vi "Lab Panel V4.87.vi"() -> ()   [LabVIEW 2013] (continued)
                          }
                          frame #9 {
                            n2885 = Greater?(x=w5378, y=w5381) -> (0:w5380:bool)
                            n2886 = case shown="True" w5380 {
                              tunnel: [w5382 0] -> w5377
                              tunnel: w5378 -> [w5382 _]
                              tunnel: w5379 -> [_ w5383]
                              frame False {
                              }
                              frame True {
                                n2887 = Concatenate Strings("LA05-2 ", w5383) -> (w5386:string)
                                n2888 = One Button Dialog(message=w5386) -> ()  [unwired: 1 in, 1 out]
                              }
                            }
                          }
                        }
                        n2889 = Bundle By Name(cluster=w5285, "LAB01-1"=w5283, "LAB01-2"=w5281, "LAB02-1"=w5278, "LAB02-2"=w5275, "LAB03-1"=w5273, "LAB03-2"=w5272, "LAB04-1"=w5269, "LAB04-2"=w5267, "LAB05-1"=w5265, "LAB05-2"=w5263) -> (w5284:T8)
                        n2890 = local write "JIG RELAY CYCLES"(w5284) -> ()
                      }
                    }
                  }
                }
              }
            }
          }
          frame #19 {
            # "get temperature values"
            n2891 = local read "PANEL #"() -> (w5387:dbl)
            n2892 = local read "simulate"() -> (w5400:bool)
            n2893 = local read "Temp Test Cal"() -> (w5397:dbl)
            n2894 = stacked-sequence {
              seq-local: [w5401 _] -> [_ w5439]
              tunnel: w5400 -> [_ w5453]
              tunnel: T14 {"1  (A) cal"=1.0, "1 (V) cal"=1.0, "1 (PF) cal"=1.0, "1 (TL) cal"=1.0, "1 (TN) cal"=1.0, "2 (A) cal"=1.0, "2 (V) cal"=1.0, "2 (PF) cal"=1.0, "2 (TL) cal"=1.0, "2 (TN) cal"=1.0} ("CAL LAB01") -> [_ w5452]
              tunnel: w5398 -> [_ w5451]
              tunnel: w5397 -> [_ w5450]
              tunnel: w5396 -> [_ w5449]
              tunnel: w5395 -> [_ w5448]
              tunnel: w5394 -> [_ w5447]
              tunnel: w5393 -> [_ w5446]
              tunnel: w5392 -> [_ w5445]
              tunnel: w5391 -> [_ w5444]
              tunnel: w5390 -> [_ w5443]
              tunnel: w5389 -> [_ w5442]
              tunnel: w5388 -> [_ w5441]
              tunnel: w5387 -> [_ w5440]
              frame #0 {
                n2895 = local read "Select COM port"() -> (w5404:refnum<visa-resource-name>)
                "COM port" <- w5404
                n2896 = global write "Global 1.vi" "tmp dly lps"("Temp Delay Lps") -> ()
                n2897 = global write "Global 1.vi" "dly value"("Temp Value") -> ()
                n2898 = global write "Global 1.vi" "COM port"(w5404) -> ()
                n2899 = local read "jig cycle"() -> (w5406:dbl)
                n2900 = local read "on loops"() -> (w5408:dbl)
                n2901 = Add(x=w5408, y=3) -> (x+y=w5409:dbl)
                n2902 = local read "PANEL #"() -> (w5405:dbl)
                n2903 = Equal?(x=w5406, y=w5409) -> (x = y?=w5401:bool)
                n2904 = case shown="True" w5401 {
                  tunnel: w5405 -> [_ w5413]
                  frame False {
                  }
                  frame True {
                    n2905 = local read "simulate"() -> (w5410:bool)
                    n2906 = case shown="1" w5413 {
                      tunnel: 1.0 -> [_ w5418 w5420 w5426 w5430 w5435]
                      tunnel: w5410 -> [_ w5414 w5419 w5424 w5431 w5434]
                      frame 0, Default {
                      }
                      frame 1 {
                        w5416 = FALSE
                        n2907 = call "sub vi - GET ALL TEMP v6.vi"("LA01-EN"=TRUE, "simulate"=w5414, "LA02-EN"=w5416, "LA03-EN"=w5416, "LA04-EN"=w5416, "LA05-EN"=w5416, "Gen Cal Value"=w5418) -> ("LA01 TEMP"=w5415:T24)  [unwired: 3 in, 5 out]
                        n2908 = local write "LAB01 TEMP"(w5415) -> ()
                      }
                      frame 2 {
                        w5421 = FALSE
                        n2909 = call "sub vi - GET ALL TEMP v6.vi"("LA01-EN"=w5421, "simulate"=w5419, "LA02-EN"=TRUE, "LA03-EN"=w5421, "LA04-EN"=w5421, "LA05-EN"=w5421, "Gen Cal Value"=w5420) -> ("LA02 TEMP"=w5423:T24)  [unwired: 3 in, 5 out]
                        n2910 = local write "LAB02 TEMP"(w5423) -> ()
                      }
                      frame 3 {
                        w5427 = FALSE
                        n2911 = call "sub vi - GET ALL TEMP v6.vi"("LA01-EN"=w5427, "simulate"=w5424, "LA02-EN"=w5427, "LA03-EN"=TRUE, "LA04-EN"=w5427, "LA05-EN"=w5427, "Gen Cal Value"=w5426) -> ("LA03 TEMP"=w5425:T24)  [unwired: 3 in, 5 out]
                        n2912 = local write "LAB03 TEMP"(w5425) -> ()
                      }
                      frame 4 {
                        w5432 = FALSE
                        n2913 = call "sub vi - GET ALL TEMP v6.vi"("LA01-EN"=w5432, "simulate"=w5431, "LA02-EN"=w5432, "LA03-EN"=w5432, "LA04-EN"=TRUE, "LA05-EN"=w5432, "Gen Cal Value"=w5430) -> ("LA04 TEMP"=w5429:T24)  [unwired: 3 in, 5 out]
                        n2914 = local write "LAB04 TEMP"(w5429) -> ()
                      }
                      frame 5 {
                        w5437 = FALSE
                        n2915 = call "sub vi - GET ALL TEMP v6.vi"("LA01-EN"=w5437, "simulate"=w5434, "LA02-EN"=w5437, "LA03-EN"=w5437, "LA04-EN"=w5437, "LA05-EN"=TRUE, "Gen Cal Value"=w5435) -> ("LA05 TEMP"=w5436:T24)  [unwired: 3 in, 5 out]
                        n2916 = local write "LAB05 TEMP"(w5436) -> ()
                      }
                    }
                    n2917 = local write "TEMP"(TRUE) -> ()
                  }
                }
              }
              frame #1 {
                n2918 = case shown="True" w5439 {
                  tunnel: w5453 -> [_ w5467]
                  tunnel: w5452 -> [_ w5466]
                  tunnel: w5451 -> [_ w5465]
                  tunnel: w5450 -> [_ w5464]
                  tunnel: w5449 -> [_ w5463]
                  tunnel: w5448 -> [_ w5462]
                  tunnel: w5447 -> [_ w5461]
                  tunnel: w5446 -> [_ w5460]
                  tunnel: w5445 -> [_ w5459]
                  tunnel: w5444 -> [_ w5458]
                  tunnel: w5443 -> [_ w5457]
                  tunnel: w5442 -> [_ w5456]
                  tunnel: w5441 -> [_ w5455]
                  tunnel: w5440 -> [_ w5454]
                  frame False {
                  }
                  frame True {
                    n2919 = case shown="1" w5454 {
                      tunnel: w5467 -> [_ w5480 w5525 w5570 w5615 w5660]
                      tunnel: w5466 -> [_ w5479 w5524 w5569 w5614 w5659]
                      tunnel: w5465 -> [_ w5477 _ _ _ _]
                      tunnel: w5464 -> [_ w5473 w5523 w5568 w5613 w5658]
                      tunnel: w5463 -> [_ w5468 _ _ _ _]
                      tunnel: w5462 -> [_ _ w5514 _ _ _]
                      tunnel: w5461 -> [_ _ w5513 _ _ _]
                      tunnel: w5460 -> [_ _ _ w5559 _ _]
                      tunnel: w5459 -> [_ _ _ w5558 _ _]
                      tunnel: w5458 -> [_ _ _ _ w5604 _]
                      tunnel: w5457 -> [_ _ _ _ w5603 _]
                      tunnel: w5456 -> [_ _ _ _ _ w5649]
                      tunnel: w5455 -> [_ _ _ _ _ w5648]
                      frame ..0 {
                      }
                      frame 1 {
                        n2920 = case shown="False" w5480 {
                          tunnel: [w5511 w5512] -> w5496
                          tunnel: w5479 -> [_ w5512]
                          frame False {
                            n2921 = local read "CAL LAB01"() -> (w5511:T14)
                          }
                          frame True {
                          }
                        }
                        n2922 = local read "LAB01 TEMP"() -> (w5486:T12)
                        n2923 = local read "TEMP LA01"() -> (w5487:T9)
                        n2924 = call "sub vi - temperature delay v2.vi"("temp values IN"=w5487, "temp signals"=w5486) -> ("T2-N"=w5482:dbl, "T2-L"=w5483:dbl, "T1-N"=w5484:dbl, "T1-L"=w5485:dbl, "temp values OUT"=w5481:T43)  [unwired: 5 in]
                        n2925 = Unbundle By Name(w5496) -> ("1 (TL) cal"=w5491:dbl, "1 (TN) cal"=w5490:dbl, "2 (TL) cal"=w5489:dbl, "2 (TN) cal"=w5488:dbl)  [unwired: 6 out]
                        n2926 = local write "TEMP LA01"(w5481) -> ()
                        n2927 = Multiply(x=w5485, y=w5491) -> (x*y=w5478:dbl)
                        n2928 = Multiply(x=w5484, y=w5490) -> (x*y=w5475:dbl)
                        n2929 = Multiply(x=w5483, y=w5489) -> (x*y=w5472:dbl)
                        n2930 = Multiply(x=w5482, y=w5488) -> (x*y=w5471:dbl)
                        n2931 = case shown="True" w5477 {
                          tunnel: w5478 -> [w5505 w5510]
                          tunnel: w5473 -> [_ w5508]
                          tunnel: [w5505 w5509] -> w5476
                          tunnel: w5475 -> [w5504 w5507]
                          tunnel: [w5504 w5506] -> w5474
                          frame False {
                          }
                          frame True {
                            n2932 = Multiply(x=w5508, y=w5507) -> (x*y=w5506:dbl)
                            n2933 = Multiply(x=w5508, y=w5510) -> (x*y=w5509:dbl)
                          }
                        }
                        n2934 = case shown="True" w5468 {
                          tunnel: w5472 -> [w5498 w5503]
                          tunnel: w5473 -> [_ w5501]
                          tunnel: [w5498 w5502] -> w5470
                          tunnel: w5471 -> [w5497 w5500]
                          tunnel: [w5497 w5499] -> w5469
                          frame False {
                          }
                          frame True {
                            n2935 = Multiply(x=w5501, y=w5500) -> (x*y=w5499:dbl)
                            n2936 = Multiply(x=w5501, y=w5503) -> (x*y=w5502:dbl)
                          }
                        }
                        n2937 = local read "SIG LAB01-2"() -> (w5493:T2)
                        n2938 = local read "SIG LAB01-1"() -> (w5495:T2)
                        n2939 = Bundle By Name(cluster=w5495, "Tmp Live"=w5476, "Tmp Neut"=w5474) -> (w5494:T2)
                        n2940 = Bundle By Name(cluster=w5493, "Tmp Live"=w5470, "Tmp Neut"=w5469) -> (w5492:T2)
                        n2941 = local write "SIG LAB01-1"(w5494) -> ()
                        n2942 = local write "SIG LAB01-2"(w5492) -> ()
                      }
                      frame 2 {
                        n2943 = case shown="True" w5525 {
                          tunnel: [w5556 w5557] -> w5541
                          tunnel: w5524 -> [_ w5557]
                          frame False {
                            n2944 = local read "CAL LAB02"() -> (w5556:T15)
                          }
                          frame True {
                          }
                        }
                        n2945 = local read "LAB02 TEMP"() -> (w5532:T12)
                        n2946 = local read "TEMP LA02"() -> (w5531:T9)
                        n2947 = call "sub vi - temperature delay v2.vi"("temp values IN"=w5531, "temp signals"=w5532) -> ("T2-N"=w5526:dbl, "T2-L"=w5527:dbl, "T1-N"=w5528:dbl, "T1-L"=w5529:dbl, "temp values OUT"=w5530:T43)  [unwired: 5 in]
                        n2948 = Unbundle By Name(w5541) -> ("1 (TL) cal"=w5536:dbl, "1 (TN) cal"=w5535:dbl, "2 (TL) cal"=w5534:dbl, "2 (TN) cal"=w5533:dbl)  [unwired: 6 out]
                        n2949 = local write "TEMP LA02"(w5530) -> ()
                        n2950 = Multiply(x=w5529, y=w5536) -> (x*y=w5522:dbl)
                        n2951 = Multiply(x=w5528, y=w5535) -> (x*y=w5521:dbl)
                        n2952 = Multiply(x=w5527, y=w5534) -> (x*y=w5518:dbl)
                        n2953 = Multiply(x=w5526, y=w5533) -> (x*y=w5517:dbl)
                        n2954 = case shown="True" w5514 {
                          tunnel: w5522 -> [w5550 w5555]
                          tunnel: w5523 -> [_ w5553]
                          tunnel: [w5550 w5554] -> w5520
                          tunnel: w5521 -> [w5549 w5552]
                          tunnel: [w5549 w5551] -> w5519
                          frame False {
                          }
                          frame True {
                            n2955 = Multiply(x=w5553, y=w5552) -> (x*y=w5551:dbl)
                            n2956 = Multiply(x=w5553, y=w5555) -> (x*y=w5554:dbl)
                          }
                        }
                        n2957 = case shown="True" w5513 {
                          tunnel: w5518 -> [w5543 w5548]
                          tunnel: w5523 -> [_ w5546]
                          tunnel: [w5543 w5547] -> w5516
                          tunnel: w5517 -> [w5542 w5545]
                          tunnel: [w5542 w5544] -> w5515
                          frame False {
                          }
                          frame True {
                            n2958 = Multiply(x=w5546, y=w5545) -> (x*y=w5544:dbl)
                            n2959 = Multiply(x=w5546, y=w5548) -> (x*y=w5547:dbl)
                          }
                        }
                        n2960 = local read "SIG LAB02-2"() -> (w5538:T2)
                        n2961 = local read "SIG LAB02-1"() -> (w5540:T2)
                        n2962 = Bundle By Name(cluster=w5540, "Tmp Live"=w5520, "Tmp Neut"=w5519) -> (w5539:T2)
                        n2963 = Bundle By Name(cluster=w5538, "Tmp Live"=w5516, "Tmp Neut"=w5515) -> (w5537:T2)
                        n2964 = local write "SIG LAB02-1"(w5539) -> ()
                        n2965 = local write "SIG LAB02-2"(w5537) -> ()
                      }
                      frame 3 {
                        n2966 = case shown="False" w5570 {
                          tunnel: [w5601 w5602] -> w5586
                          tunnel: w5569 -> [_ w5602]
                          frame False {
                            n2967 = local read "CAL LAB03"() -> (w5601:T14)
                          }
                          frame True {
                          }
                        }
                        n2968 = local read "TEMP LA03"() -> (w5576:T9)
                        n2969 = local read "LAB03 TEMP"() -> (w5577:T12)
                        n2970 = call "sub vi - temperature delay v2.vi"("temp values IN"=w5576, "temp signals"=w5577) -> ("T2-N"=w5571:dbl, "T2-L"=w5572:dbl, "T1-N"=w5573:dbl, "T1-L"=w5574:dbl, "temp values OUT"=w5575:T43)  [unwired: 5 in]
                        n2971 = Unbundle By Name(w5586) -> ("1 (TL) cal"=w5581:dbl, "1 (TN) cal"=w5580:dbl, "2 (TL) cal"=w5579:dbl, "2 (TN) cal"=w5578:dbl)  [unwired: 6 out]
                        n2972 = local write "TEMP LA03"(w5575) -> ()
                        n2973 = Multiply(x=w5574, y=w5581) -> (x*y=w5567:dbl)
                        n2974 = Multiply(x=w5573, y=w5580) -> (x*y=w5566:dbl)
                        n2975 = Multiply(x=w5572, y=w5579) -> (x*y=w5563:dbl)
                        n2976 = Multiply(x=w5571, y=w5578) -> (x*y=w5562:dbl)
                        n2977 = case shown="True" w5558 {
                          tunnel: w5563 -> [w5588 w5593]
                          tunnel: w5568 -> [_ w5591]
                          tunnel: [w5588 w5592] -> w5561
                          tunnel: w5562 -> [w5587 w5590]
                          tunnel: [w5587 w5589] -> w5560
                          frame False {
                          }
                          frame True {
                            n2978 = Multiply(x=w5591, y=w5590) -> (x*y=w5589:dbl)
                            n2979 = Multiply(x=w5591, y=w5593) -> (x*y=w5592:dbl)
                          }
                        }
                        n2980 = case shown="True" w5559 {
                          tunnel: w5567 -> [w5595 w5600]
                          tunnel: w5568 -> [_ w5598]
                          tunnel: [w5595 w5599] -> w5565
                          tunnel: w5566 -> [w5594 w5597]
                          tunnel: [w5594 w5596] -> w5564
                          frame False {
                          }
                          frame True {
                            n2981 = Multiply(x=w5598, y=w5597) -> (x*y=w5596:dbl)
                            n2982 = Multiply(x=w5598, y=w5600) -> (x*y=w5599:dbl)
                          }
                        }
                        n2983 = local read "SIG LAB03-2"() -> (w5583:T2)
                        n2984 = local read "SIG LAB03-1"() -> (w5585:T2)
                        n2985 = Bundle By Name(cluster=w5585, "Tmp Live"=w5565, "Tmp Neut"=w5564) -> (w5584:T2)
                        n2986 = Bundle By Name(cluster=w5583, "Tmp Live"=w5561, "Tmp Neut"=w5560) -> (w5582:T2)
                        n2987 = local write "SIG LAB03-1"(w5584) -> ()
                        n2988 = local write "SIG LAB03-2"(w5582) -> ()
                      }
                      frame 4 {
                        n2989 = case shown="False" w5615 {
                          tunnel: [w5646 w5647] -> w5631
                          tunnel: w5614 -> [_ w5647]
                          frame False {
                            n2990 = local read "CAL LAB04"() -> (w5646:T14)
                          }
                          frame True {
                          }
                        }
                        n2991 = local read "LAB04 TEMP"() -> (w5621:T12)
                        n2992 = local read "TEMP LA04"() -> (w5622:T9)
                        n2993 = call "sub vi - temperature delay v2.vi"("temp values IN"=w5622, "temp signals"=w5621) -> ("T2-N"=w5616:dbl, "T2-L"=w5617:dbl, "T1-N"=w5618:dbl, "T1-L"=w5619:dbl, "temp values OUT"=w5620:T43)  [unwired: 5 in]
                        n2994 = Unbundle By Name(w5631) -> ("1 (TL) cal"=w5626:dbl, "1 (TN) cal"=w5625:dbl, "2 (TL) cal"=w5624:dbl, "2 (TN) cal"=w5623:dbl)  [unwired: 6 out]
                        n2995 = local write "TEMP LA04"(w5620) -> ()
                        n2996 = Multiply(x=w5619, y=w5626) -> (x*y=w5612:dbl)
                        n2997 = Multiply(x=w5618, y=w5625) -> (x*y=w5611:dbl)
                        n2998 = Multiply(x=w5617, y=w5624) -> (x*y=w5608:dbl)
                        n2999 = Multiply(x=w5616, y=w5623) -> (x*y=w5607:dbl)
                        n3000 = case shown="True" w5603 {
                          tunnel: w5608 -> [w5633 w5638]
                          tunnel: w5613 -> [_ w5636]
                          tunnel: [w5633 w5637] -> w5606
                          tunnel: w5607 -> [w5632 w5635]
                          tunnel: [w5632 w5634] -> w5605
                          frame False {
                          }
                          frame True {
                            n3001 = Multiply(x=w5636, y=w5635) -> (x*y=w5634:dbl)
                            n3002 = Multiply(x=w5636, y=w5638) -> (x*y=w5637:dbl)
                          }
                        }
                        n3003 = case shown="True" w5604 {
                          tunnel: w5612 -> [w5640 w5645]
                          tunnel: w5613 -> [_ w5643]
                          tunnel: [w5640 w5644] -> w5610
                          tunnel: w5611 -> [w5639 w5642]
                          tunnel: [w5639 w5641] -> w5609
                          frame False {
                          }
                          frame True {
                            n3004 = Multiply(x=w5643, y=w5642) -> (x*y=w5641:dbl)
                            n3005 = Multiply(x=w5643, y=w5645) -> (x*y=w5644:dbl)
                          }
                        }
                        n3006 = local read "SIG LAB04-2"() -> (w5628:T2)
                        n3007 = local read "SIG LAB04-1"() -> (w5630:T2)
                        n3008 = Bundle By Name(cluster=w5630, "Tmp Live"=w5610, "Tmp Neut"=w5609) -> (w5629:T2)
                        n3009 = Bundle By Name(cluster=w5628, "Tmp Live"=w5606, "Tmp Neut"=w5605) -> (w5627:T2)
                        n3010 = local write "SIG LAB04-1"(w5629) -> ()
                        n3011 = local write "SIG LAB04-2"(w5627) -> ()
                      }
                      frame 5.. {
                        n3012 = case shown="False" w5660 {
                          tunnel: [w5691 w5692] -> w5676
                          tunnel: w5659 -> [_ w5692]
                          frame False {
                            n3013 = local read "CAL LAB05"() -> (w5691:T14)
                          }
                          frame True {
                          }
                        }
                        n3014 = local read "LAB05 TEMP"() -> (w5666:T12)
                        n3015 = local read "TEMP LA05"() -> (w5667:T9)
                        n3016 = call "sub vi - temperature delay v2.vi"("temp values IN"=w5667, "temp signals"=w5666) -> ("T2-N"=w5662:dbl, "T2-L"=w5663:dbl, "T1-N"=w5664:dbl, "T1-L"=w5665:dbl, "temp values OUT"=w5661:T43)  [unwired: 5 in]
                        n3017 = local write "TEMP LA05"(w5661) -> ()
                        n3018 = Unbundle By Name(w5676) -> ("1 (TL) cal"=w5668:dbl, "1 (TN) cal"=w5671:dbl, "2 (TL) cal"=w5670:dbl, "2 (TN) cal"=w5669:dbl)  [unwired: 6 out]
                        n3019 = Multiply(x=w5665, y=w5668) -> (x*y=w5657:dbl)
                        n3020 = Multiply(x=w5664, y=w5671) -> (x*y=w5656:dbl)
                        n3021 = Multiply(x=w5663, y=w5670) -> (x*y=w5653:dbl)
                        n3022 = Multiply(x=w5662, y=w5669) -> (x*y=w5652:dbl)
                        n3023 = case shown="True" w5648 {
                          tunnel: w5653 -> [w5678 w5683]
                          tunnel: w5658 -> [_ w5681]
                          tunnel: [w5678 w5682] -> w5651
                          tunnel: w5652 -> [w5677 w5680]
                          tunnel: [w5677 w5679] -> w5650
                          frame False {
                          }
                          frame True {
                            n3024 = Multiply(x=w5681, y=w5680) -> (x*y=w5679:dbl)
                            n3025 = Multiply(x=w5681, y=w5683) -> (x*y=w5682:dbl)
                          }
                        }
                        n3026 = case shown="True" w5649 {
                          tunnel: w5657 -> [w5685 w5690]
                          tunnel: w5658 -> [_ w5688]
                          tunnel: [w5685 w5689] -> w5655
                          tunnel: w5656 -> [w5684 w5687]
                          tunnel: [w5684 w5686] -> w5654
                          frame False {
                          }
                          frame True {
                            n3027 = Multiply(x=w5688, y=w5687) -> (x*y=w5686:dbl)
                            n3028 = Multiply(x=w5688, y=w5690) -> (x*y=w5689:dbl)
                          }
                        }
                        n3029 = local read "SIG LAB05-1"() -> (w5675:T2)
                        n3030 = Bundle By Name(cluster=w5675, "Tmp Live"=w5655, "Tmp Neut"=w5654) -> (w5674:T2)
                        n3031 = local read "SIG LAB05-2"() -> (w5673:T2)
                        n3032 = Bundle By Name(cluster=w5673, "Tmp Live"=w5651, "Tmp Neut"=w5650) -> (w5672:T2)
                        n3033 = local write "SIG LAB05-1"(w5674) -> ()
                        n3034 = local write "SIG LAB05-2"(w5672) -> ()
                      }
                    }
                  }
                }
              }
            }
          }
          frame #20 {
            # "write data to display panel"
            n3035 = global write "Global display 1.vi" "TEST 5-2"(w5727) -> ()
            n3036 = global write "Global display 1.vi" "TEST 4-2"(w5729) -> ()
            n3037 = global write "Global display 1.vi" "TEST 1-2"(w5735) -> ()
            n3038 = global write "Global display 1.vi" "TEST 3-1"(w5732) -> ()
            n3039 = global write "Global display 1.vi" "TEST 5-1"(w5728) -> ()
            n3040 = global write "Global display 1.vi" "TEST 1-1"(w5736) -> ()
            n3041 = global write "Global display 1.vi" "TEST 3-2"(w5731) -> ()
            n3042 = global write "Global display 1.vi" "TEST 4-1"(w5730) -> ()
            n3043 = global write "Global display 1.vi" "TEST 2-2"(w5733) -> ()
            n3044 = global write "Global display 1.vi" "TEST 2-1"(w5734) -> ()
            n3045 = global read "Global display 3.vi" "log 1-1"() -> (→"LOG LAB01-1":string)
            n3046 = global read "Global display 3.vi" "log 3-1"() -> (→"LOG LAB03-1":string)
            n3047 = global read "Global display 3.vi" "log 1-2"() -> (→"LOG LAB01-2":string)
            n3048 = property on="Tab Control 2" class="TabCtl (strict)"() -> ("Pages"=w5726:refnum<vi>[])  [unwired: 2 in, 2 out]
            n3049 = global read "Global display 3.vi" "log 2-1"() -> (→"LOG LAB02-1":string)
            n3050 = global read "Global display 3.vi" "log 2-2"() -> (→"LOG LAB02-2":string)
            n3051 = global read "Global display 3.vi" "log 4-2"() -> (→"LOG LAB04-2":string)
            n3052 = global read "Global display 3.vi" "log 5-2"() -> (→"LOG LAB05-2":string)
            n3053 = global read "Global display 3.vi" "log 5-1"() -> (→"LOG LAB05-1":string)
            n3054 = global read "Global display 3.vi" "log 4-1"() -> (→"LOG LAB04-1":string)
            n3055 = global read "Global display 3.vi" "log 3-2"() -> (→"LOG LAB03-2":string)
            n3056 = Index Array(array=w5726, index=9) -> (element=w5724:refnum<vi>)
            n3057 = property class="Page"(reference=w5724) -> ("PageVis"=w5723:bool)  [unwired: 1 in, 2 out]
            n3058 = global write "Global display 3.vi" "admin"(w5723) -> ()
            n3059 = local read "O/I  LAB05-2"() -> (w5777:bool)
            n3060 = local read "O/I  LAB05-1"() -> (w5778:bool)
            n3061 = local read "O/I  LAB03-2"() -> (w5781:bool)
            n3062 = local read "O/I  LAB04-2"() -> (w5779:bool)
            n3063 = local read "O/I  LAB04-1"() -> (w5780:bool)
            n3064 = local read "O/I  LAB03-1"() -> (w5782:bool)
            n3065 = local read "O/I  LAB01-2"() -> (w5785:bool)
            n3066 = local read "O/I  LAB01-1"() -> (w5786:bool)
            n3067 = local read "O/I  LAB02-1"() -> (w5784:bool)
            n3068 = local read "O/I  LAB02-2"() -> (w5783:bool)
            n3069 = global write "Global display 1.vi" "5-2 O/F"(w5777) -> ()
            n3070 = global write "Global display 1.vi" "5-1 O/F"(w5778) -> ()
            n3071 = global write "Global display 1.vi" "4-1 O/F"(w5780) -> ()
            n3072 = global write "Global display 1.vi" "4-2 O/F"(w5779) -> ()
            n3073 = global write "Global display 1.vi" "3-2 O/F"(w5781) -> ()
            n3074 = global write "Global display 1.vi" "3-1 O/F"(w5782) -> ()
            n3075 = global write "Global display 1.vi" "2-2 O/F"(w5783) -> ()
            n3076 = global write "Global display 1.vi" "2-1 O/F"(w5784) -> ()
            n3077 = global write "Global display 1.vi" "1-2 O/F"(w5785) -> ()
            n3078 = global write "Global display 1.vi" "1-1 O/F"(w5786) -> ()
            n3079 = local read "TEMP START LAB02-2"() -> (w5709:cluster{"TL":dbl, "TN":dbl})
            n3080 = local read "run lab05-2"() -> (w5767:bool)
            n3081 = local read "TEMP START LAB01-2"() -> (w5711:cluster{"TL":dbl, "TN":dbl})
            n3082 = local read "TEMP START LAB02-1"() -> (w5710:cluster{"TL":dbl, "TN":dbl})
            n3083 = local read "TEMP START LAB04-1"() -> (w5706:cluster{"TL":dbl, "TN":dbl})
            n3084 = local read "TEMP START LAB04-2"() -> (w5705:cluster{"TL":dbl, "TN":dbl})
            n3085 = local read "run lab04-1"() -> (w5770:bool)
            n3086 = local read "run lab04-2"() -> (w5769:bool)
            n3087 = local read "run lab05-1"() -> (w5768:bool)
            n3088 = local read "TEMP START LAB01-1"() -> (w5712:cluster{"TL":dbl, "TN":dbl})
            n3089 = local read "TEMP START LAB05-2"() -> (w5703:cluster{"TL":dbl, "TN":dbl})
            n3090 = local read "TEMP START LAB05-1"() -> (w5704:cluster{"TL":dbl, "TN":dbl})
            n3091 = local read "run lab03-2"() -> (w5771:bool)
            n3092 = local read "TEMP START LAB03-2"() -> (w5707:cluster{"TL":dbl, "TN":dbl})
            n3093 = local read "TEMP START LAB03-1"() -> (w5708:cluster{"TL":dbl, "TN":dbl})
            n3094 = local read "run lab02-1"() -> (w5774:bool)
            n3095 = local read "run lab03-1"() -> (w5772:bool)
            n3096 = local read "run lab01-2"() -> (w5775:bool)
            n3097 = local read "run lab02-2"() -> (w5773:bool)
            n3098 = local read "run lab01-1"() -> (w5776:bool)
            n3099 = global write "Global display 1.vi" "5-2 R/S"(w5767) -> ()
            n3100 = global write "Global display 1.vi" "5-1 R/S"(w5768) -> ()
            n3101 = global write "Global display 1.vi" "4-2 R/S"(w5769) -> ()
            n3102 = global write "Global display 1.vi" "4-1 R/S"(w5770) -> ()
            n3103 = global write "Global display 1.vi" "3-2 R/S"(w5771) -> ()
            n3104 = global write "Global display 1.vi" "1-2 R/S"(w5775) -> ()
            n3105 = global write "Global display 1.vi" "2-1 R/S"(w5774) -> ()
            n3106 = global write "Global display 1.vi" "3-1 R/S"(w5772) -> ()
            n3107 = global write "Global display 1.vi" "2-2 R/S"(w5773) -> ()
            n3108 = global write "Global display 1.vi" "1-1 R/S"(w5776) -> ()
            n3109 = global write "Global display 3.vi" "TEMP ST 05-2"(w5703) -> ()
            n3110 = global write "Global display 3.vi" "TEMP ST 05-1"(w5704) -> ()
            n3111 = global write "Global display 3.vi" "TEMP ST 03-2"(w5707) -> ()
            n3112 = global write "Global display 3.vi" "TEMP ST 04-2"(w5705) -> ()
            n3113 = global write "Global display 3.vi" "TEMP ST 01-1"(w5712) -> ()
            n3114 = global write "Global display 3.vi" "TEMP ST 01-2"(w5711) -> ()
            n3115 = global write "Global display 3.vi" "TEMP ST 04-1"(w5706) -> ()
            n3116 = global write "Global display 3.vi" "TEMP ST 02-1"(w5710) -> ()
            n3117 = global write "Global display 3.vi" "TEMP ST 02-2"(w5709) -> ()
            n3118 = global write "Global display 3.vi" "TEMP ST 03-1"(w5708) -> ()
            n3119 = local read "DISP LAB04-2"() -> (w5759:T4)
            n3120 = local read "DISP LAB05-1"() -> (w5758:T4)
            n3121 = local read "DISP LAB04-1"() -> (w5760:T4)
            n3122 = local read "DISP LAB05-2"() -> (w5757:T4)
            n3123 = local read "DISP LAB03-1"() -> (w5762:T4)
            n3124 = local read "DISP LAB03-2"() -> (w5761:T4)
            n3125 = local read "DISP LAB01-2"() -> (w5765:T4)
            n3126 = local read "DISP LAB02-1"() -> (w5764:T4)
            n3127 = local read "DISP LAB02-2"() -> (w5763:T4)
            n3128 = local read "DISP LAB01-1"() -> (w5766:T4)
            n3129 = local read "TEMP RISE LAB05-1"() -> (w5694:cluster{"TL":dbl, "TN":dbl})
            n3130 = local read "TEMP RISE LAB05-2"() -> (w5693:cluster{"TL":dbl, "TN":dbl})
            n3131 = local read "TEMP RISE LAB04-2"() -> (w5695:cluster{"TL":dbl, "TN":dbl})
            n3132 = local read "TEMP RISE LAB04-1"() -> (w5696:cluster{"TL":dbl, "TN":dbl})
            n3133 = local read "TEMP RISE LAB03-2"() -> (w5697:cluster{"TL":dbl, "TN":dbl})
            n3134 = local read "TEMP RISE LAB03-1"() -> (w5698:cluster{"TL":dbl, "TN":dbl})
            n3135 = local read "TEMP RISE LAB01-2"() -> (w5701:cluster{"TL":dbl, "TN":dbl})
            n3136 = local read "TEMP RISE LAB02-2"() -> (w5699:cluster{"TL":dbl, "TN":dbl})
            n3137 = local read "TEMP RISE LAB01-1"() -> (w5702:cluster{"TL":dbl, "TN":dbl})
            n3138 = local read "TEMP RISE LAB02-1"() -> (w5700:cluster{"TL":dbl, "TN":dbl})
            n3139 = global write "Global display 2.vi" "DISP LAB05-1"(w5758) -> ()
            n3140 = global write "Global display 2.vi" "DISP LAB05-2"(w5757) -> ()
            n3141 = global write "Global display 2.vi" "DISP LAB04-2"(w5759) -> ()
            n3142 = global write "Global display 2.vi" "DISP LAB02-1"(w5764) -> ()
            n3143 = global write "Global display 2.vi" "DISP LAB02-2"(w5763) -> ()
            n3144 = global write "Global display 2.vi" "DISP LAB04-1"(w5760) -> ()
            n3145 = global write "Global display 2.vi" "DISP LAB01-2"(w5765) -> ()
            n3146 = global write "Global display 2.vi" "DISP LAB01-1"(w5766) -> ()
            n3147 = global write "Global display 2.vi" "DISP LAB03-1"(w5762) -> ()
            n3148 = global write "Global display 2.vi" "DISP LAB03-2"(w5761) -> ()
            n3149 = global write "Global display 3.vi" "TEMP RS 05-2"(w5693) -> ()
            n3150 = global write "Global display 3.vi" "TEMP RS 05-1"(w5694) -> ()
            n3151 = global write "Global display 3.vi" "TEMP RS 03-2"(w5697) -> ()
            n3152 = global write "Global display 3.vi" "TEMP RS 02-1"(w5700) -> ()
            n3153 = global write "Global display 3.vi" "TEMP RS 02-2"(w5699) -> ()
            n3154 = global write "Global display 3.vi" "TEMP RS 04-2"(w5695) -> ()
            n3155 = global write "Global display 3.vi" "TEMP RS 01-2"(w5701) -> ()
            n3156 = global write "Global display 3.vi" "TEMP RS 03-1"(w5698) -> ()
            n3157 = global write "Global display 3.vi" "TEMP RS 04-1"(w5696) -> ()
            n3158 = global write "Global display 3.vi" "TEMP RS 01-1"(w5702) -> ()
            n3159 = local read "SET LAB05-2"() -> (w5747:T5)
            n3160 = local read "SET LAB05-1"() -> (w5748:T5)
            n3161 = local read "SET LAB04-1"() -> (w5750:T5)
            n3162 = local read "SET LAB04-2"() -> (w5749:T5)
            n3163 = local read "SET LAB03-1"() -> (w5752:T5)
            n3164 = local read "SET LAB03-2"() -> (w5751:T5)
            n3165 = local read "SET LAB02-2"() -> (w5753:T5)
            n3166 = local read "SET LAB01-2"() -> (w5755:T5)
            n3167 = local read "SET LAB02-1"() -> (w5754:T5)
            n3168 = local read "SET LAB01-1"() -> (w5756:T5)
            n3169 = global write "Global display 2.vi" "SET LAB05-2"(w5747) -> ()
            n3170 = global write "Global display 2.vi" "SET LAB05-1"(w5748) -> ()
            n3171 = global write "Global display 2.vi" "SET LAB04-1"(w5750) -> ()
            n3172 = global write "Global display 2.vi" "SET LAB04-2"(w5749) -> ()
            n3173 = global write "Global display 2.vi" "SET LAB03-2"(w5751) -> ()
            n3174 = global write "Global display 2.vi" "SET LAB02-2"(w5753) -> ()
            n3175 = global write "Global display 2.vi" "SET LAB03-1"(w5752) -> ()
            n3176 = global write "Global display 2.vi" "SET LAB01-2"(w5755) -> ()
            n3177 = global write "Global display 2.vi" "SET LAB01-1"(w5756) -> ()
            n3178 = global write "Global display 2.vi" "SET LAB02-1"(w5754) -> ()
            n3179 = local read "RESULT LAB01-1"() -> (w5746:bool)
            n3180 = local read "RESULT LAB03-2"() -> (w5741:bool)
            n3181 = local read "RESULT LAB04-1"() -> (w5740:bool)
            n3182 = local read "RESULT LAB04-2"() -> (w5739:bool)
            n3183 = local read "RESULT LAB02-2"() -> (w5743:bool)
            n3184 = local read "RESULT LAB01-2"() -> (w5745:bool)
            n3185 = local read "RESULT LAB02-1"() -> (w5744:bool)
            n3186 = local read "RESULT LAB03-1"() -> (w5742:bool)
            n3187 = local read "RESULT LAB05-1"() -> (w5738:bool)
            n3188 = local read "RESULT LAB05-2"() -> (w5737:bool)
            n3189 = global write "Global display 2.vi" "RESULT LAB05-1"(w5738) -> ()
            n3190 = global write "Global display 2.vi" "RESULT LAB01-2"(w5745) -> ()
            n3191 = global write "Global display 2.vi" "RESULT LAB03-2"(w5741) -> ()
            n3192 = global write "Global display 2.vi" "RESULT LAB04-1"(w5740) -> ()
            n3193 = global write "Global display 2.vi" "RESULT LAB04-2"(w5739) -> ()
            n3194 = global write "Global display 2.vi" "RESULT LAB05-2"(w5737) -> ()
            n3195 = global write "Global display 2.vi" "RESULT LAB03-1"(w5742) -> ()
            n3196 = global write "Global display 2.vi" "RESULT LAB02-1"(w5744) -> ()
            n3197 = global write "Global display 2.vi" "RESULT LAB02-2"(w5743) -> ()
            n3198 = global write "Global display 2.vi" "RESULT LAB01-1"(w5746) -> ()
          }
          frame #21 {
            # "simulate values"
            n3199 = global write "Global display 4.vi" "LAB deg C"("LAB deg C") -> ()
          }
          frame #22 {
            # "end main and display program"
            n3200 = Quit LabVIEW(quit? (T)="stop all") -> ()
            n3201 = global write "Global display 1.vi" "stop disp"("stop all") -> ()
          }
        }
        n3202 = node-c288() -> ()  [unwired: 1 in, 1 out]
        "loops" <- w297
      }
      n3203 = node-c288(w274) -> ()  [unwired: 1 out]
    }
  }
